vi "Example Threshold.vi"() -> ()   [LabVIEW 2013]
uses:
  C:/tf/play/labview/Tinkerforge.dll
  Tinkerforge.dll
panel:
  in  "stop":bool
  out "callback counter":i32
  out "last voltage (V)":sgl
  in  "uid":string="amb"
  in  "port":i32=4223
  in  "host":string="localhost"
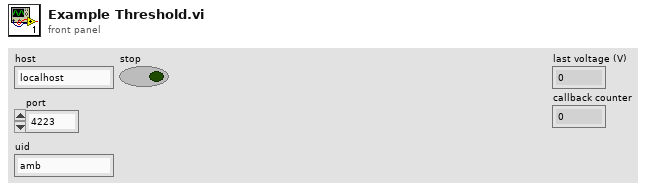
[diagram p1: front panel]
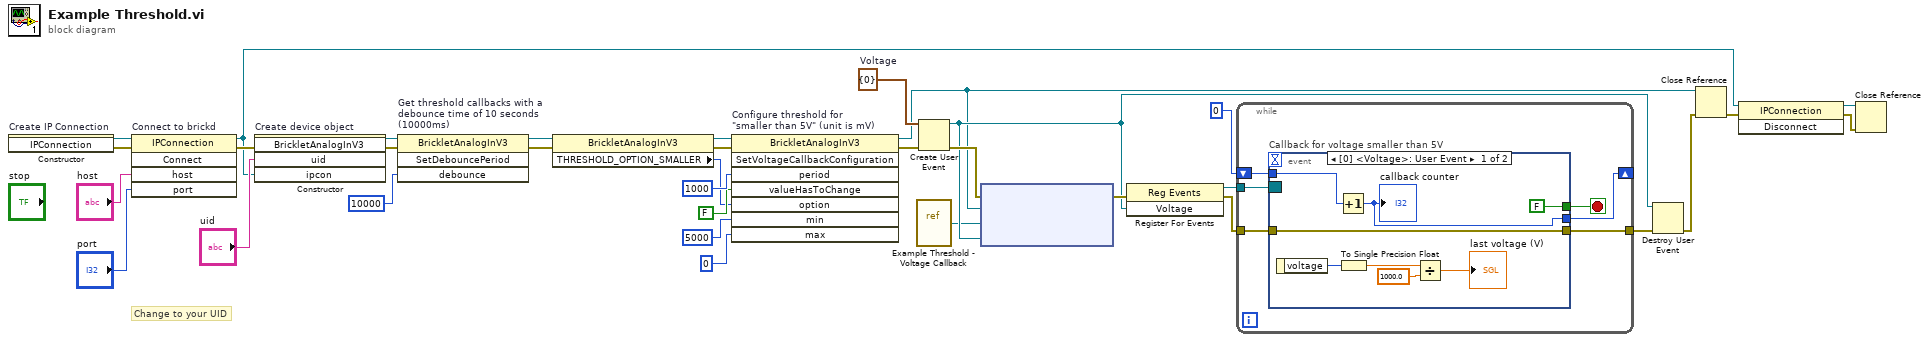
[diagram p0: block diagram]
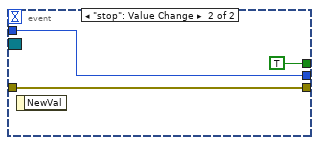
[diagram p2: hidden frame]
diagram:
  w18 = cluster{"voltage":i32} {"voltage"=0}  # Voltage
  # "Change to your UID"
  n1 = constructor on="Create IP Connection" class="IPConnection"() -> (reference out=w34:refnum<k24>, error out=w7:errorcluster)  [unwired: 3 in, 1 out]
  n2 = invoke on="Connect to brickd" class="IPConnection" method="Connect"(reference=w34, error in=w7, "host"="host", "port"="port") -> (reference out=w27:refnum<k24>, error out=w30:errorcluster)  [unwired: 1 in, 3 out]
  n3 = constructor on="Create device object" class="BrickletAnalogInV3"(error in=w30, "uid"="uid", "ipcon"=w27) -> (reference out=w16:refnum<k24>, error out=w17:errorcluster)  [unwired: 2 in, 3 out]
  n4 = invoke on="Get threshold callbacks with a\ndebounce time of 10 seconds\n(10000ms)" class="BrickletAnalogInV3" method="SetDebouncePeriod"(reference=w16, error in=w17, "debounce"=i64 10000 ("period")) -> (reference out=w10:refnum<k24>, error out=w12:errorcluster)  [unwired: 1 in, 2 out]
  n5 = property class="BrickletAnalogInV3"(reference=w10, error in=w12) -> (reference out=w9:refnum<k24>, error out=w11:errorcluster, "THRESHOLD_OPTION_SMALLER"=w4:u16)
  n6 = invoke on="Configure threshold for\n\"smaller than 5V\" (unit is mV)" class="BrickletAnalogInV3" method="SetVoltageCallbackConfiguration"(reference=w9, error in=w11, "period"=i64 1000, "valueHasToChange"=FALSE, "option"=w4, "min"=5000, "max"=0) -> (reference out=w14:refnum<k24>, error out=w13:errorcluster)  [unwired: 1 in, 6 out]
  n7 = vi-ref "Example Threshold - Voltage Callback.vi"() -> ("vi reference"=w1:refnum<vi>)
  n8 = Create User Event(user event datatype=w18, error in=w13) -> (user event=w20:refnum<user-event>, error out=w25:errorcluster)
  n9 = node ("Register Event Callback")(w25, w14, w1, w20) -> (w24:errorcluster)  [unwired: 1 in, 1 out]
  n10 = register-events(error in=w24, w20) -> (reference out=w23:refnum<event-registration>, error out=w21:errorcluster)  [unwired: 1 in]
  n11 = while {
    tunnel: w23 -> [w40]
    tunnel: [w39] -> w22
    tunnel: w21 -> [w38]
    shift-right: [w36] -> _
    shift-left: 0 -> [w37]
    stop <- w35 stop-if-true
    n12 = event "Callback for voltage smaller than 5V" shown="[0] <Voltage>: User Event" {
      selector: w40 -> [_ _]
      dyn-events: _ -> [_ _]
      timeout: _ -> [_ _]
      tunnel: [w45 w50] -> w39
      tunnel: w38 -> [w45 w50]
      tunnel: w37 -> [w43 w49]
      tunnel: [w42 w49] -> w36
      tunnel: [FALSE TRUE] -> w35
      event User Event {
        n13 = event-data() -> ("voltage"=w46:i32)  [unwired: 1 in]
        n14 = Increment(x=w43) -> (x+1=w42:i32)
        "callback counter" <- w42
        n15 = To Single Precision Float(number=w46) -> (single precision float=w47:sgl)
        n16 = Divide(x=w47, y=sgl 1000.0) -> (x/y=→"last voltage (V)":sgl)
      }
      event "stop": Value Change {
        n17 = event-data() -> ()  [unwired: 1 in, 1 out]
      }
    }
  }
  n18 = Destroy User Event(user event=w20, error in=w22) -> (error out=w19:errorcluster)
  n19 = Close Reference(reference=w14, error in (no error)=w19) -> (error out=w29:errorcluster)
  n20 = invoke class="IPConnection" method="Disconnect"(reference=w27, error in=w29) -> (reference out=w26:refnum<k24>, error out=w28:errorcluster)  [unwired: 1 in, 1 out]
  n21 = Close Reference(reference=w26, error in (no error)=w28) -> ()  [unwired: 1 out]
